vi "Set Item Data.vi"(8 "error in (no error)":errorcluster, 10 "Front Panel Controls":T1, 11 "VI in":refnum<class "VI.lvclass">) -> (0 "error out":errorcluster, 3 "VI out":refnum<class "VI.lvclass">)   [LabVIEW 2020, in "VI Properties Editor.lvlib" / "VI.lvclass"]
doc: "Sets the values of <B>Front Panel Controls</B> to the values of the data of <B>VI in</B>."
uses:
  VI.lvclass
  CTLs/Main Front Panel Controls.ctl
  Item/Item.lvclass
  VI Properties Editor.lvlib
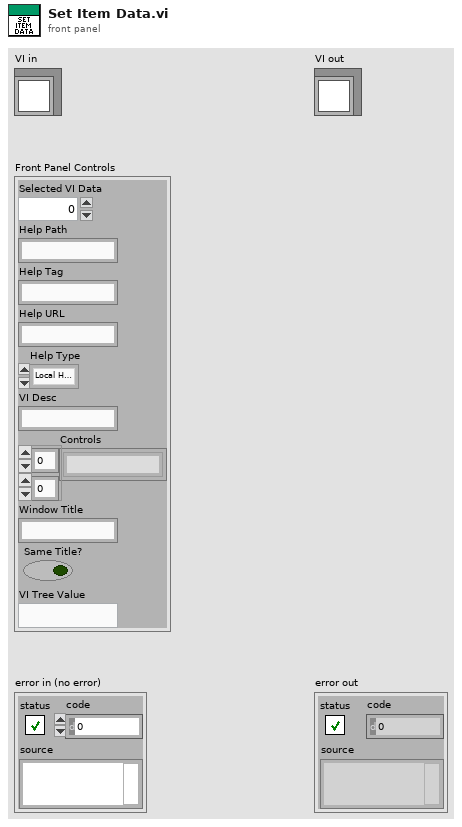
[diagram p1: front panel]
types:
  T1 = typedef "VI Properties Editor.lvlib/Main Front Panel Controls.ctl" = cluster{"Selected VI Data":i32, "Help Path":string, "Help Tag":string, "Help URL":string, "Help Type":enum16{"Local Help File", "Web-based Help"}, "VI Desc":string, "Controls":string[][], "Window Title":string, "Same Title?":bool, "VI Tree Value":string}
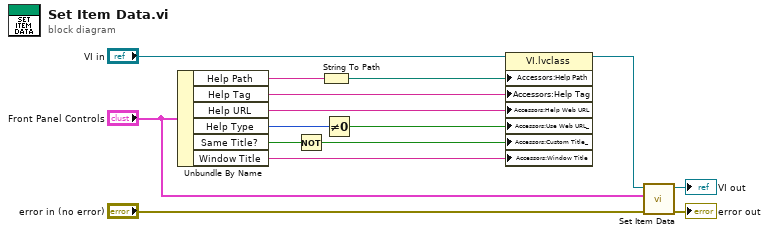
[diagram p0: block diagram]
diagram:
  n1 = Unbundle By Name("Front Panel Controls") -> ("Help Path"=w9:string, "Help Tag"=w7:string, "Help URL"=w6:string, "Help Type"=w5:enum16{"Local Help File", "Web-based Help"}, "Same Title?"=w3:bool, "Window Title"=w1:string)
  n2 = Not(x=w3) -> (.not. x?=w2:bool)
  n3 = String To Path(string=w9) -> (path=w8:path)
  n4 = Not Equal To 0?(x=w5) -> (x != 0?=w4:bool)
  n5 = property class="VI.lvclass"(reference="VI in", "Accessors:Help Path"=w8, "Accessors:Help Tag"=w7, "Accessors:Help Web URL"=w6, "Accessors:Use Web URL_"=w4, "Accessors:Custom Title_"=w2, "Accessors:Window Title"=w1) -> (reference out=w11:refnum<class "VI.lvclass">)  [unwired: 1 in, 1 out]
  n6 = call-parent "Set Item Data.vi"("error in (no error)"="error in (no error)", "Front Panel Controls"="Front Panel Controls", "Item in"=w11) -> ("error out"=→"error out":errorcluster, "Item out"=→"VI out":refnum<class "VI.lvclass">)  [unwired: 7 in]
